vi "Mouse Zoom.vi"(7 "PlatMods":T1, 8 "error in (no error)":errorcluster, 9 "XY":cluster{"X":dbl, "Y":dbl}, 10 "Delta":i32, 11 "XY Graph":refnum<vi>) -> ()   [LabVIEW 2020, in "Graph Extensions.lvlib"]
doc: "Zooming works for several areas:\n\n1. No modifiers, just straight scroll wheel. This zooms on the X-Axis to zoom in and out\n2. SHIFT, changes the zoom to be on the Y-Axis\n3. CTRL, changes to a pan mode, sliding on the X-Axis with the scroll wheel\n4. CTRL SHIFT, pans on the Y-Axis with the scroll wheel"
uses:
  Graph Extensions.lvlib
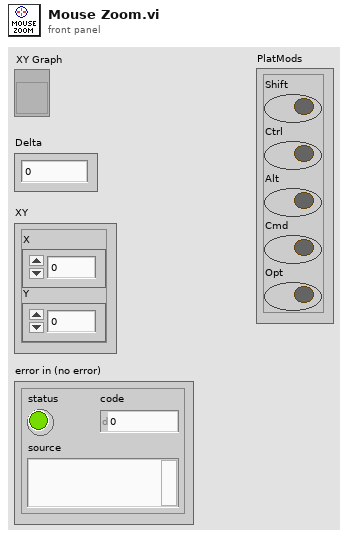
[diagram p1: front panel]
types:
  T1 = cluster{"Shift":bool, "Ctrl":bool, "Alt":bool, "Cmd":bool, "Opt":bool}
  T2 = typedef "LVRectTypeDef.ctl" = cluster{"Left":i16, "Top":i16, "Right":i16, "Bottom":i16}
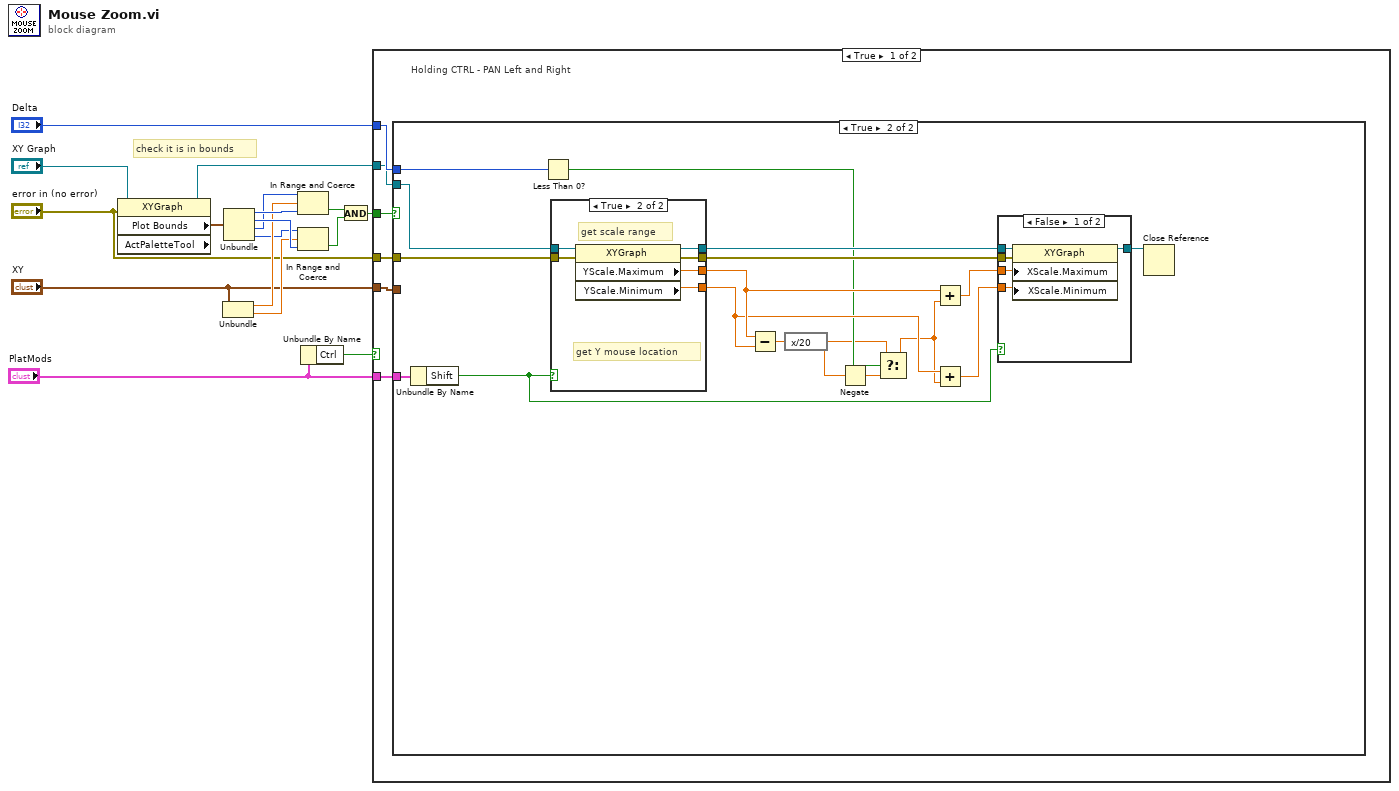
[diagram p0: block diagram]
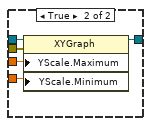
[diagram p3: hidden frame]
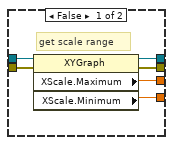
[diagram p4: hidden frame]
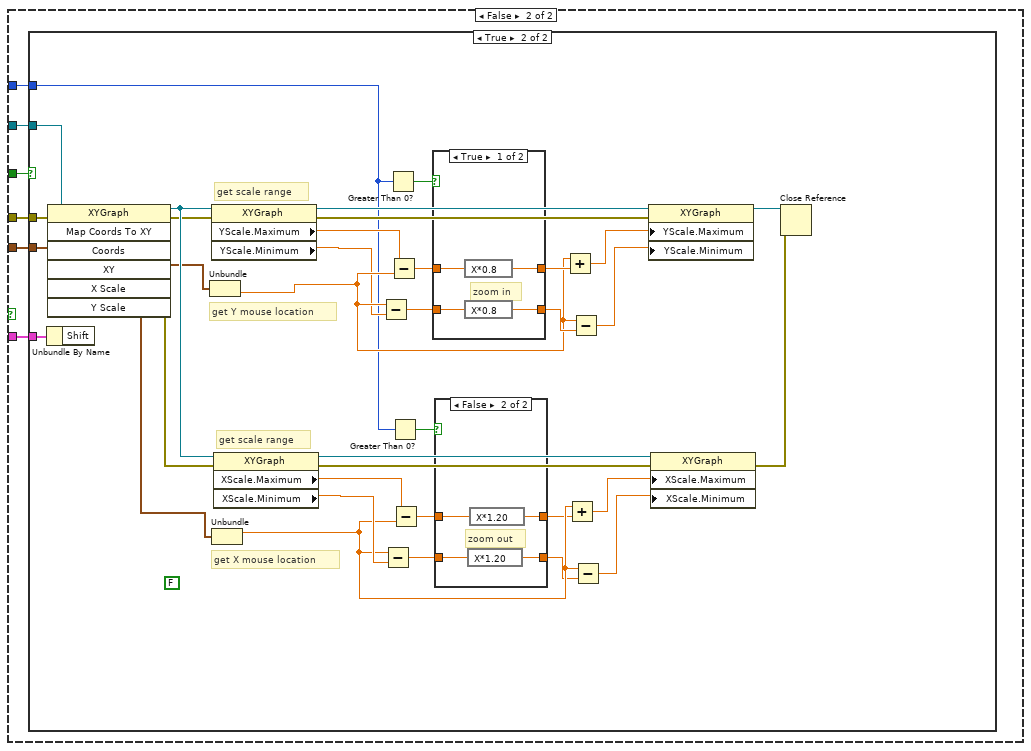
[diagram p5: hidden frame]
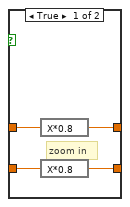
[diagram p7: hidden frame]
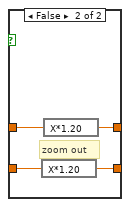
[diagram p8: hidden frame]
diagram:
  # "check it is in bounds"
  n1 = property on="Property Node" class="XYGraph" props=["Plot Bounds", "ActPaletteTool"](reference="XY Graph", error in="error in (no error)") -> (reference out=w3:refnum<vi>, "Plot Bounds"=w6:T2)  [unwired: 2 out]
  n2 = Unbundle("XY") -> ("X"=w13:dbl, "Y"=w14:dbl)
  n3 = Unbundle(w6) -> ("Left"=w16:i16, "Top"=w15:i16, "Right"=w12:i16, "Bottom"=w11:i16)
  n4 = In Range and Coerce(upper limit=w12, x=w13, lower limit=w16) -> (In Range?=w10:bool)  [unwired: 1 out]
  n5 = In Range and Coerce(upper limit=w11, x=w14, lower limit=w15) -> (In Range?=w9:bool)  [unwired: 1 out]
  n6 = Unbundle By Name("PlatMods") -> ("Ctrl"=w1:bool)
  n7 = And(x=w10, y=w9) -> (x .and. y?=w4:bool)
  n8 = case shown="True" w1 {
    tunnel: "Delta" -> [w23 w68]
    tunnel: "error in (no error)" -> [w22 w67]
    tunnel: "XY" -> [w21 w66]
    tunnel: w4 -> [w20 w65]
    tunnel: w3 -> [w19 w64]
    tunnel: "PlatMods" -> [w18 w63]
    frame True {
      # "Holding CTRL - PAN Left and Right"
      n9 = case shown="True" w20 {
        tunnel: w23 -> [_ w36]
        tunnel: w19 -> [_ w32]
        tunnel: w22 -> [_ w31]
        tunnel: w21 -> [_ _]
        tunnel: w18 -> [_ w34]
        frame False {
          # "not in the plot range, so ignore the scroll wheel"
        }
        frame True {
          n10 = Unbundle By Name(w34) -> ("Shift"=w33:bool)
          n11 = Less Than 0?(x=w36) -> (x < 0?=w27:bool)
          n12 = case shown="True" w33 {
            tunnel: [w56 w62] -> w29
            tunnel: [w55 w61] -> w28
            tunnel: [w54 w60] -> w38
            tunnel: [w53 w59] -> w37
            tunnel: w31 -> [w52 w58]
            tunnel: w32 -> [w51 w57]
            frame False {
              # "get scale range"
              n13 = property on="Property Node" class="XYGraph"(reference=w51, error in=w52) -> (reference out=w53:refnum<vi>, error out=w54:errorcluster, "XScale.Maximum"=w56:dbl, "XScale.Minimum"=w55:dbl)
            }
            frame True {
              # "get scale range"
              # "get Y mouse location"
              n14 = property on="Property Node" class="XYGraph"(reference=w57, error in=w58) -> (reference out=w59:refnum<vi>, error out=w60:errorcluster, "YScale.Maximum"=w62:dbl, "YScale.Minimum"=w61:dbl)
            }
          }
          n15 = Subtract(x=w29, y=w28) -> (x-y=w30:dbl)
          n16 = expression code="x/20"(w30) -> (w24:dbl)
          n17 = Negate(x=w24) -> (-x=w26:dbl)
          n18 = Select(t=w24, s=w27, f=w26) -> (s? t:f=w25:dbl)
          n19 = Add(x=w29, y=w25) -> (x+y=w39:dbl)
          n20 = Add(x=w28, y=w25) -> (x+y=w40:dbl)
          n21 = case shown="False" w33 {
            tunnel: w40 -> [w41 w50]
            tunnel: w39 -> [w42 w49]
            tunnel: w38 -> [w44 w48]
            tunnel: w37 -> [w45 w47]
            tunnel: [w43 w46] -> w35
            frame False {
              n22 = property on="Property Node" class="XYGraph"(reference=w45, error in=w44, "XScale.Maximum"=w42, "XScale.Minimum"=w41) -> (reference out=w43:refnum<vi>)  [unwired: 1 out]
            }
            frame True {
              n23 = property on="Property Node" class="XYGraph"(reference=w47, error in=w48, "YScale.Maximum"=w49, "YScale.Minimum"=w50) -> (reference out=w46:refnum<vi>)  [unwired: 1 out]
            }
          }
          n24 = Close Reference(reference=w35) -> ()  [unwired: 1 in, 1 out]
        }
      }
    }
    frame False {
      n25 = case shown="True" w65 {
        tunnel: w68 -> [_ w73]
        tunnel: w64 -> [_ w96]
        tunnel: w67 -> [_ w95]
        tunnel: w66 -> [_ w94]
        tunnel: w63 -> [_ w93]
        frame False {
          # "not in the plot range, so ignore the scroll wheel"
        }
        frame True {
          (unwired) FALSE
          # "get scale range"
          # "get Y mouse location"
          # "get scale range"
          # "get X mouse location"
          n26 = Unbundle By Name(w93) -> ()  [unwired: 1 out]
          n27 = invoke on="Invoke Node" class="XYGraph" method="Map Coords To XY"(reference=w96, error in=w95, "Coords"=w94) -> (reference out=w72:refnum<vi>, error out=w71:errorcluster, "XY"=w70:cluster{"X":dbl, "Y":dbl})  [unwired: 4 in, 4 out]
          n28 = Unbundle(w70) -> ("Y"=w88:dbl)  [unwired: 1 out]
          n29 = property on="Property Node" class="XYGraph"(reference=w72, error in=w71) -> (reference out=w99:refnum<vi>, error out=w100:errorcluster, "YScale.Maximum"=w90:dbl, "YScale.Minimum"=w87:dbl)
          n30 = Unbundle(w70) -> ("X"=w83:dbl)  [unwired: 1 out]
          n31 = property on="Property Node" class="XYGraph"(reference=w72, error in=w71) -> (reference out=w77:refnum<vi>, error out=w76:errorcluster, "XScale.Maximum"=w81:dbl, "XScale.Minimum"=w84:dbl)
          n32 = Subtract(x=w88, y=w87) -> (x-y=w86:dbl)
          n33 = Subtract(x=w83, y=w84) -> (x-y=w85:dbl)
          n34 = Greater Than 0?(x=w73) -> (x > 0?=w98:bool)
          n35 = Subtract(x=w90, y=w88) -> (x-y=w89:dbl)
          n36 = Greater Than 0?(x=w73) -> (x > 0?=w78:bool)
          n37 = Subtract(x=w81, y=w83) -> (x-y=w82:dbl)
          n38 = case shown="True" w98 {
            tunnel: w89 -> [w114 w118]
            tunnel: [w113 w117] -> w101
            tunnel: w86 -> [w112 w116]
            tunnel: [w111 w115] -> w92
            frame True {
              # "zoom in"
              n39 = expression code="X*0.8"(w114) -> (w113:dbl)
              n40 = expression code="X*0.8"(w112) -> (w111:dbl)
            }
            frame False {
              # "zoom out"
              n41 = expression code="X*1.20"(w116) -> (w115:dbl)
              n42 = expression code="X*1.20"(w118) -> (w117:dbl)
            }
          }
          n43 = case shown="False" w78 {
            tunnel: w82 -> [w106 w110]
            tunnel: [w105 w109] -> w75
            tunnel: w85 -> [w104 w108]
            tunnel: [w103 w107] -> w79
            frame True {
              # "zoom in"
              n44 = expression code="X*0.8"(w106) -> (w105:dbl)
              n45 = expression code="X*0.8"(w104) -> (w103:dbl)
            }
            frame False {
              # "zoom out"
              n46 = expression code="X*1.20"(w108) -> (w107:dbl)
              n47 = expression code="X*1.20"(w110) -> (w109:dbl)
            }
          }
          n48 = Add(x=w88, y=w101) -> (x+y=w102:dbl)
          n49 = Add(x=w83, y=w75) -> (x+y=w74:dbl)
          n50 = Subtract(x=w88, y=w92) -> (x-y=w91:dbl)
          n51 = Subtract(x=w83, y=w79) -> (x-y=w80:dbl)
          n52 = property on="Property Node" class="XYGraph"(reference=w99, error in=w100, "YScale.Maximum"=w102, "YScale.Minimum"=w91) -> (reference out=w97:refnum<vi>)  [unwired: 1 out]
          n53 = property on="Property Node" class="XYGraph"(reference=w77, error in=w76, "XScale.Maximum"=w74, "XScale.Minimum"=w80) -> (error out=w69:errorcluster)  [unwired: 1 out]
          n54 = Close Reference(reference=w97, error in (no error)=w69) -> ()  [unwired: 1 out]
        }
      }
    }
  }
